vi "Spin Shooter (Auto).vi"(10 "RPM (1900)":dbl=1900.0, 11 "Execute?":bool) -> (2 "Numeric":i32, 3 "Done":bool)   [LabVIEW 2012]
uses:
  <vilib>/addons/control/pid/pid.llb/PID (DBL).vi
  <vilib>/addons/control/pid/NI_PID_pid.lvlib
panel:
  out "Motor Out":dbl
  in  "Shooter Wheel PID gains":T1={"proportional gain (Kc)"=0.03, "integral time (Ti, min)"=0.0, "derivative time (Td, min)"=0.0} {"derivative time (Td, min)" format="%.3f"; "integral time (Ti, min)" format="%.3f"; "proportional gain (Kc)" format="%.3f"}
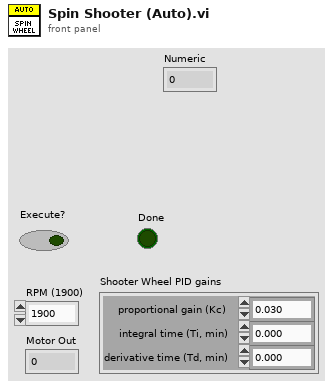
[diagram p1: front panel]
types:
  T1 = cluster{"proportional gain (Kc)":dbl, "integral time (Ti, min)":dbl, "derivative time (Td, min)":dbl}
  T2 = typedef "WPI_CounterDevRef.ctl" = cluster{"DevStatus":errorcluster, "CntIndex":T3}
  T3 = typedef "FPGA_CounterCtrSystemIndex.ctl" = enum8{"Ctr 0", "Ctr 1", "Ctr 2", "Ctr 3", "Ctr 4", "Ctr 5", "Ctr 6", "Ctr 7", "Invalid"}
  T4 = typedef "WPI_MotorControlDeviceRef.ctl" = cluster{"DeviceStatus":errorcluster, "Type":enum16{"PWM", "CAN"}, "PWM":cluster{"Digital Module":T5, "PWM Channel":T6, "DeadBand":T7}, "CAN":cluster{"Device Number":u8, "Control Mode":T8, "Semaphore":T9, "Max Vout":dbl}, "Invert":bool, "TransformRef":T10, "InvTransformRef":T10}
  T5 = typedef "FPGA_TypedefDigitalModule.ctl" = enum16{"Digital Module 1", "Digital Module 2"}
  T6 = typedef "FPGA_DIOPWMChannel.ctl" = enum8{"PWM 1", "PWM 2", "PWM 3", "PWM 4", "PWM 5", "PWM 6", "PWM 7", "PWM 8", "PWM 9", "PWM 10", "Invalid"}
  T7 = typedef "WPI_PWMDeadband.ctl" = cluster{"Name":string, "maxPositivePwm":i32, "minPositivePwm":i32, "centerPwm":i32, "maxNegativePwm":i32, "minNegativePwm":i32, "angularRange":u16}
  T8 = typedef "WPI_CANJaguar_ControlMode.ctl" = enum8{"Percent VBus", "Current", "Speed", "Position", "Voltage"}
  T9 = typedef "Semaphore RefNum" = refnum<k1>
  T10 = typedef "WPI_PWMTransform_ConPane.ctl" = refnum<vi>
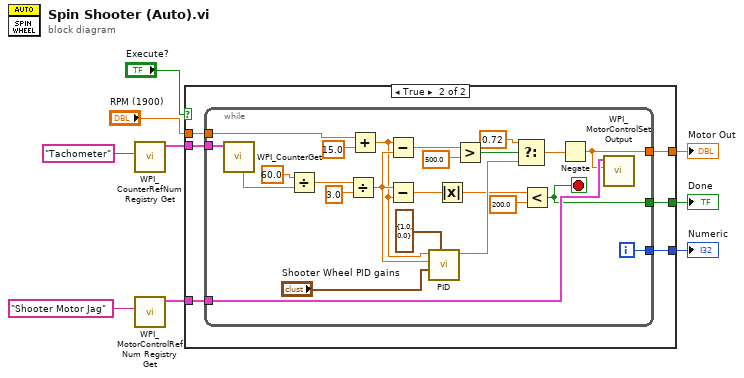
[diagram p0: block diagram]
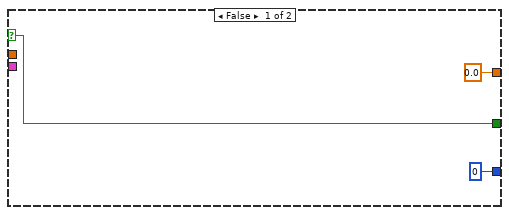
[diagram p2: hidden frame]
diagram:
  n1 = call <vilib>:"WPI_CounterRefNum Registry Get.vi"("refnum name"="Tachometer") -> ("CounterDevRef"=w3:T2)  [unwired: 9 in, 1 out]
  n2 = call <vilib>:"WPI_MotorControlRefNum Registry Get.vi"("refnum name"="Shooter Motor Jag") -> ("MotorControlDevRef"=w1:T4)  [unwired: 9 in, 1 out]
  n3 = case shown="True" "Execute?" {
    selector: "Execute?" -> [w12 _]
    tunnel: [w12 w18] -> w9
    tunnel: [0.0 w17] -> w7
    tunnel: w3 -> [_ w16]
    tunnel: "RPM (1900)" -> [_ w15]
    tunnel: w1 -> [_ w14]
    tunnel: [0 w13] -> w5
    frame False {
    }
    frame True {
      n4 = while {
        tunnel: w16 -> [w38]
        tunnel: w14 -> [w36]
        tunnel: [w24] -> w18
        tunnel: [w32] -> w17
        tunnel: w15 -> [w27]
        tunnel: [w20] -> w13
        i -> [w20]
        stop <- w24 stop-if-true
        n5 = call <vilib>:"WPI_CounterGet.vi"("CounterDevRef in"=w38) -> ("Period (sec)"=w40:dbl)  [unwired: 5 in, 5 out]
        n6 = Divide(x=60.0, y=w40) -> (x/y=w42:dbl)
        n7 = Divide(x=w42, y=3.0) -> (x/y=w26:dbl)
        n8 = Add(x=w27, y=15.0) -> (x+y=w25:dbl)
        n9 = Subtract(x=w25, y=w26) -> (x-y=w29:dbl)
        n10 = Subtract(x=w26, y=w25) -> (x-y=w22:dbl)
        n11 = call-poly <vilib>:"PID.vi"("output range"=cluster{"output high":dbl, "output low":dbl} {"output high"=1.0, "output low"=0.0}, "PID gains"="Shooter Wheel PID gains", "process variable"=w26, "setpoint"=w25) -> ("output"=w34:dbl)  [unwired: 6 in, 1 out]
        n12 = Absolute Value(x=w22) -> (abs(x)=w21:dbl)
        n13 = Greater?(x=w29, y=500.0) -> (0:w31:bool)
        n14 = Select(t=0.72, s=w31, f=w34) -> (s? t:f=w33:dbl)
        n15 = Less?(x=w21, y=200.0) -> (x < y?=w24:bool)
        n16 = Negate(x=w33) -> (-x=w32:dbl)
        n17 = call <vilib>:"WPI_MotorControlSetOutput.vi"("Output"=w32, "MotorControlDevRef"=w36) -> ()  [unwired: 7 in, 3 out]
      }
    }
  }
  "Done" <- w9
  "Motor Out" <- w7
  "Numeric" <- w5
